vi "Write Temperature to Cooler.vi"(8 "error in (no error)":errorcluster, 11 "CCDCamera in":refnum<class "CCDCamera.lvclass">) -> (0 "error out":errorcluster, 3 "CCDCamera out":refnum<class "CCDCamera.lvclass">)   [LabVIEW 2018, in "CCDCamera.lvclass"]
uses:
  CCDCamera.lvclass
  Cooler/Cooler.lvclass
  LV2018/Interface/Interface.lvclass
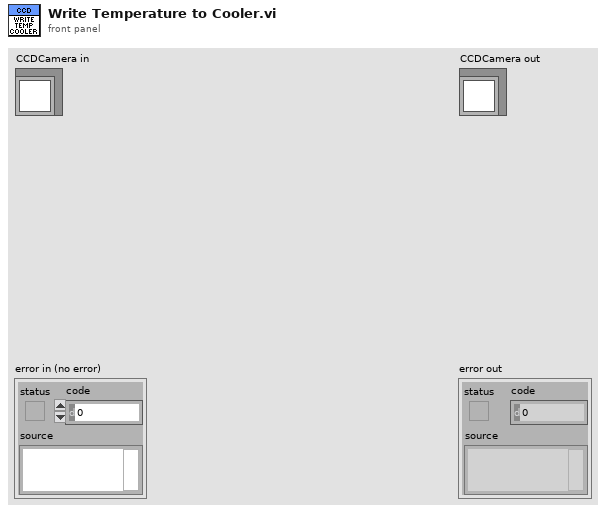
[diagram p1: front panel]
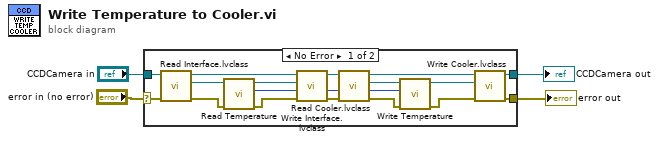
[diagram p0: block diagram]
diagram:
  n1 = case shown="No Error" "error in (no error)" {
    selector: "error in (no error)" -> [w21 w23]
    tunnel: [w9 w23] -> w3
    tunnel: [w10 w22] -> w1
    tunnel: "CCDCamera in" -> [w20 w22]
    frame No Error {
      n2 = call-dynamic "Read Interface.lvclass.vi"("error in (no error)"=w21, "CCDCamera in"=w20) -> ("error out"=w8:errorcluster, "Interface.lvclass"=w18:refnum<class "Interface.lvclass">, "CCDCamera out"=w16:refnum<class "CCDCamera.lvclass">)  [unwired: 7 in]
      n3 = call-dynamic "Read Temperature.vi"("error in (no error)"=w8, "Interface in"=w18) -> ("error out"=w7:errorcluster, "Temperature"=w19:i8, "Interface out"=w17:refnum<class "Interface.lvclass">)  [unwired: 7 in]
      n4 = call-dynamic "Write Interface.lvclass.vi"("error in (no error)"=w7, "Interface.lvclass"=w17, "CCDCamera in"=w16) -> ("error out"=w15:errorcluster, "CCDCamera out"=w14:refnum<class "CCDCamera.lvclass">)  [unwired: 7 in]
      n5 = call-dynamic "Read Cooler.lvclass.vi"("error in (no error)"=w15, "CCDCamera in"=w14) -> ("error out"=w6:errorcluster, "Cooler.lvclass"=w13:refnum<class "Cooler.lvclass">, "CCDCamera out"=w11:refnum<class "CCDCamera.lvclass">)  [unwired: 7 in]
      n6 = call-dynamic "Write Temperature.vi"("error in (no error)"=w6, "Temperature"=w19, "Cooler in"=w13) -> ("error out"=w5:errorcluster, "Cooler out"=w12:refnum<class "Cooler.lvclass">)  [unwired: 7 in]
      n7 = call-dynamic "Write Cooler.lvclass.vi"("error in (no error)"=w5, "Cooler.lvclass"=w12, "CCDCamera in"=w11) -> ("error out"=w9:errorcluster, "CCDCamera out"=w10:refnum<class "CCDCamera.lvclass">)  [unwired: 7 in]
    }
    frame Error {
    }
  }
  "error out" <- w3
  "CCDCamera out" <- w1
